vi "Conveyer Belt Process.vi"(0 "error in":errorcluster) -> ()   [LabVIEW 2012]
uses:
  Conveyer Belt Global Data.vi
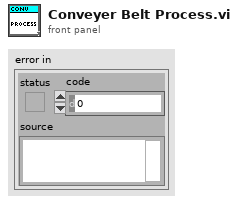
[diagram p1: front panel]
types:
  T1 = cluster{"MS Bottom":bool, "MS Middle":bool, "MS Flipper":bool, "Motor Value":dbl}
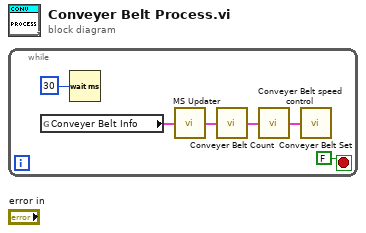
[diagram p0: block diagram]
diagram:
  n1 = while {
    stop <- FALSE stop-if-true
    n2 = global read "Conveyer Belt Global Data.vi" "Conveyer Belt Info"() -> (w5:T1)
    n3 = Wait (ms)(milliseconds to wait=u32 30) -> ()  [unwired: 1 out]
    n4 = call "MS Updater.vi"("Conveyer Belt Info"=w5) -> ("Conveyer Belt Info out"=w3:T1)
    n5 = call "Conveyer Belt Count.vi"("Conveyer Belt Info"=w3) -> ("Conveyer Belt Info Out"=w2:T1)
    n6 = call "Conveyer Belt speed control.vi"("Conveyer Belt Info"=w2) -> ("Conveyer Belt Info out"=w6:T1)
    n7 = call "Conveyer Belt Set.vi"("Conveyer Belt Info"=w6) -> ()
  }
